vi "Address2Coordinate.vi"(1 "Address":string) -> (0 "Coordinate":i32[](array[numeric]))   [LabVIEW 2026, in "XCel Report Engine.lvlib"]
uses:
  XCel Report Engine.lvlib
  C:/Users/m.santucci/Documents/ChatGPT/LV_REPORT_ENGINE/LV/DotNet/XCelReportEngine.dll
  DotNet/XCelReportEngine.dll
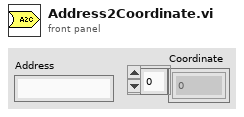
[diagram p1: front panel]
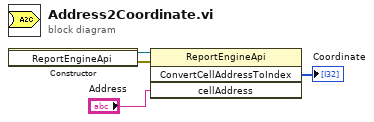
[diagram p0: block diagram]
diagram:
  n1 = constructor class="ReportEngineApi"() -> (reference out=w4:refnum<k24>, error out=w3:errorcluster)  [unwired: 3 in, 1 out]
  n2 = invoke class="ReportEngineApi" method="ConvertCellAddressToIndex"(reference=w4, error in=w3, "cellAddress"="Address") -> ("ConvertCellAddressToIndex"=→"Coordinate":i32[])  [unwired: 1 in, 3 out]
